vi "TODO Ping.vi"(0 "Client.lvclass in":refnum<class "Client.lvclass">, 11 "error in (no error)":errorcluster) -> (4 "Client.lvclass out":refnum<class "Client.lvclass">, 6 "Ping status":string, 15 "error out":errorcluster)   [LabVIEW 2018, in "InfluxDB Client.lvlib" / "Client.lvclass"]
doc: "Performs a ping to retrieve status information."
uses:
  Client.lvclass
  Client.lvclass/Client.ctl
  <vilib>/LVH/i3 JSON/JSON Parsing/Get Object Parameter Files/Get Object Parameter - String.vi
  <vilib>/httpClient/LabVIEWHTTPClient.lvlib
  <vilib>/LVH/i3 JSON/i3-json.lvlib
panel:
  out "Status":string
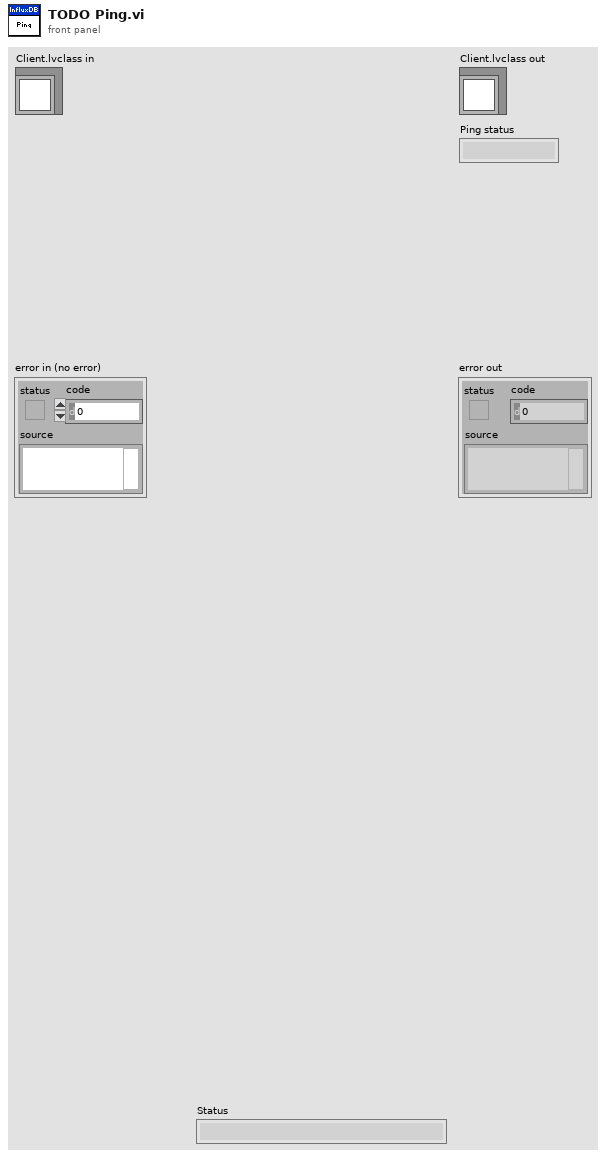
[diagram p1: front panel]
types:
  T1 = typedef "LabVIEWHTTPClient.lvlib/ClientHandle.ctl" = refnum<k1>
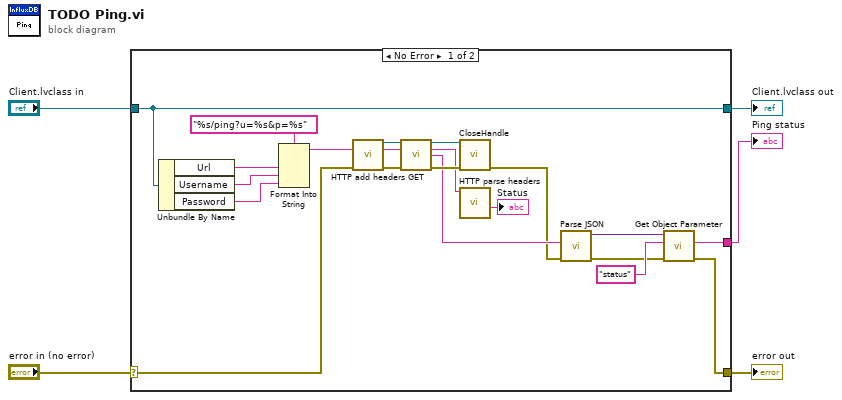
[diagram p0: block diagram]
diagram:
  n1 = case shown="No Error" "error in (no error)" {
    selector: "error in (no error)" -> [w14 w27]
    tunnel: [w8 w27] -> w4
    tunnel: [w6 w26] -> w2
    tunnel: "Client.lvclass in" -> [w6 w26]
    tunnel: [w11 _] -> w1
    frame No Error {
      n2 = Unbundle By Name(w6) -> ("Url"=w24:string, "Username"=w18:string, "Password"=w17:string)
      n3 = Format Into String(format string="%s/ping?u=%s&p=%s" ("url"), w24, w18, w17) -> (resulting string=w21:string)  [unwired: 2 in, 1 out]
      n4 = call "HTTP add headers.vi"("error in (no error)"=w14) -> ("client handle out"=w16:T1, "error out"=w15:errorcluster)  [unwired: 13 in]
      n5 = call <vilib>:"GET.vi"("client handle"=w16, "url"=w21, "error in (no error)"=w15) -> ("client handle out"=w23:T1, "headers"=w20:string, "body"=w13:string, "error out"=w22:errorcluster)  [unwired: 9 in]
      n6 = call <vilib>:"CloseHandle.vi"("client handle"=w23, "error in (no error)"=w22) -> ("error out"=w7:errorcluster)  [unwired: 13 in]
      n7 = call "HTTP parse headers.vi"("HTTP headers"=w20) -> ("Status"=→"Status":string)  [unwired: 7 in, 3 out]
      n8 = call <vilib>:"Parse JSON.vi"("error in (no error)"=w7, "JSON String"=w13) -> ("error out"=w9:errorcluster, "JSON Tree"=w12:variant)  [unwired: 6 in, 2 out]
      n9 = call-poly <vilib>:"Get Object Parameter.vi"("error in (no error)"=w9, "Parameter Name"="status", "JSON Tree In (JSON Object)"=w12) -> ("error out"=w8:errorcluster, "String Value"=w11:string)  [unwired: 5 in, 2 out]
    }
    frame Error {
    }
  }
  "error out" <- w4
  "Client.lvclass out" <- w2
  "Ping status" <- w1
